vi "high_pass_filter_2nd.vi"(7 "Input":dbl format="%.2f", 13 "Corner period":dbl(slide)=10.237739663395852 scale=1.0..1000.0) -> (8 "Output":dbl format="%.2f")   [LabVIEW 2016]
doc: "Use this VI to filter a signal using 2nd order high pass filter. The difference equation is \n[y(j)-2*y(j-1)+y(j-2)] + sqrt(2)*b*[y(j)-y(j-1)] + (b^2)*y(j) = [x(j)-2*x(j-1)+x(j-2)].\n\nInputs:\nInput,\nCorner period.\nOutputs:\nOutput.\n\nMuhannad Alghamdi\nCSUSB Physics 350"
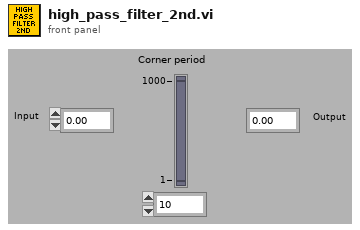
[diagram p1: front panel]
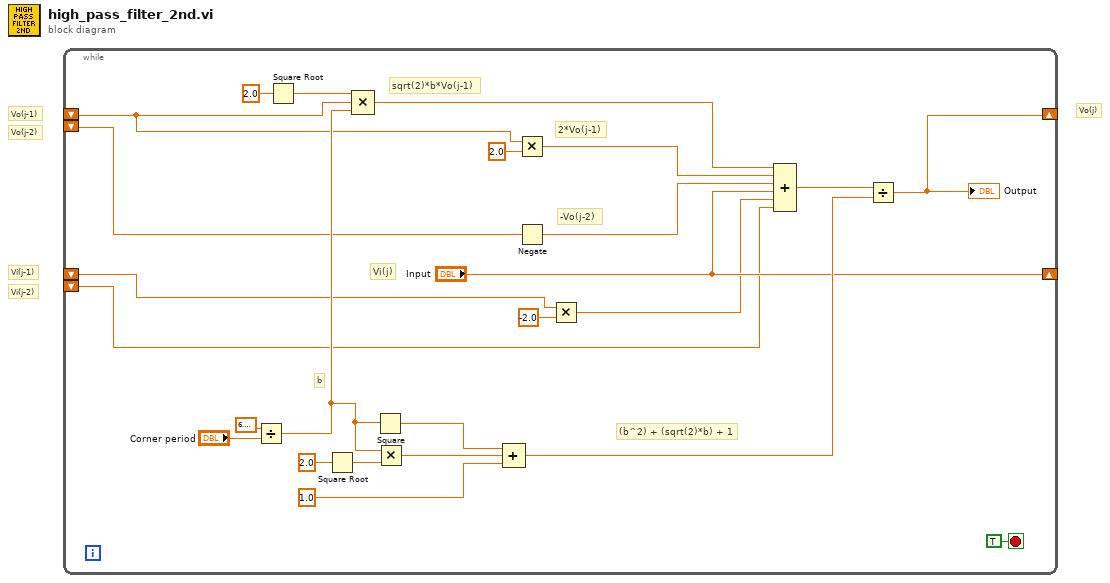
[diagram p0: block diagram]
diagram:
  # "Vi(j-1)"
  # "Vi(j-2)"
  # "Vo(j-1)"
  # "Vo(j-2)"
  # "Vo(j)"
  n1 = while {
    shift-left: _ -> [w9]
    shift-right: [w21] -> _
    shift-left: _ -> [w7]
    shift-right: ["Input"] -> _
    shift-left: _ -> [w4]
    shift-left: _ -> [w1]
    stop <- TRUE stop-if-true
    # "-Vo(j-2)"
    # "2*Vo(j-1)"
    # "sqrt(2)*b*Vo(j-1)"
    # "Vi(j)"
    # "(b^2) + (sqrt(2)*b) + 1"
    # "b"
    n2 = Divide(x=6.283185307179586, y="Corner period") -> (x/y=w11:dbl)
    n3 = Square Root(x=2.0) -> (sqrt(x)=w12:dbl)
    n4 = Square Root(x=2.0) -> (sqrt(x)=w18:dbl)
    n5 = Compound Arithmetic op=MULTIPLY(w12, w9, w11) -> (w13:dbl)
    n6 = Square(x=w11) -> (x^2=w17:dbl)
    n7 = Multiply(x=w11, y=w18) -> (x*y=w16:dbl)
    n8 = Compound Arithmetic op=ADD(w17, w16, 1.0 ("value")) -> (w20:dbl)
    n9 = Multiply(x=w9, y=2.0) -> (x*y=w8:dbl)
    n10 = Negate(x=w7) -> (-x=w6:dbl)
    n11 = Multiply(x=w4, y=-2.0) -> (x*y=w3:dbl)
    n12 = Compound Arithmetic op=ADD(w13, w8, w6, "Input", w3, w1) -> (w22:dbl)
    n13 = Divide(x=w22, y=w20) -> (x/y=w21:dbl)
    "Output" <- w21
  }
